vi "TMflexLinkInformation.vi"() -> ()   [LabVIEW 2015]
uses:
  TMflexDatabase.lvclass
  <vilib>/Utility/config.llb/Read Key (String).vi
  <vilib>/addons/database/_DB Variant To Data/Database Variant To Data.xnode
  <vilib>/Utility/config.llb/NI_LVConfig.lvlib
panel:
  out "User Name":string
  in  "Unlink Assembly":T1(radio)=enum."FinalAssembly"
  out "Sql Query":string
  in  "Reset":bool
  out "Link Table":string[][](table)
  in  "Get Link Info":bool
  in  "Stop Button":bool
  in  "Update Link Info":bool
  in  "ExtAssembly":string
  in  "PowerSupply":string
  in  "ChemicalTrap":string
  in  "OxygenSensor":string
  in  "HydrogenSensor":string
  in  "GcAssembly":string
  in  "OcAssembly":string
  in  "PasAssembly":string
  in  "QtmsAssembly":string
  in  "FinalAssembly":string
  # "TMflexLinkInfo: Tools for getting link info, linking and de-linking TMxflex assemblies\nGet Link Info: Scan in the serial number of the desired assembly and click Get Link button\nLink Assembly: Scan in serial numbers of assemblies and click Update Link button\nDe-Link Assembly: Select the unlink radio button and then click Update Link button\nQuit: Hit Stop button"
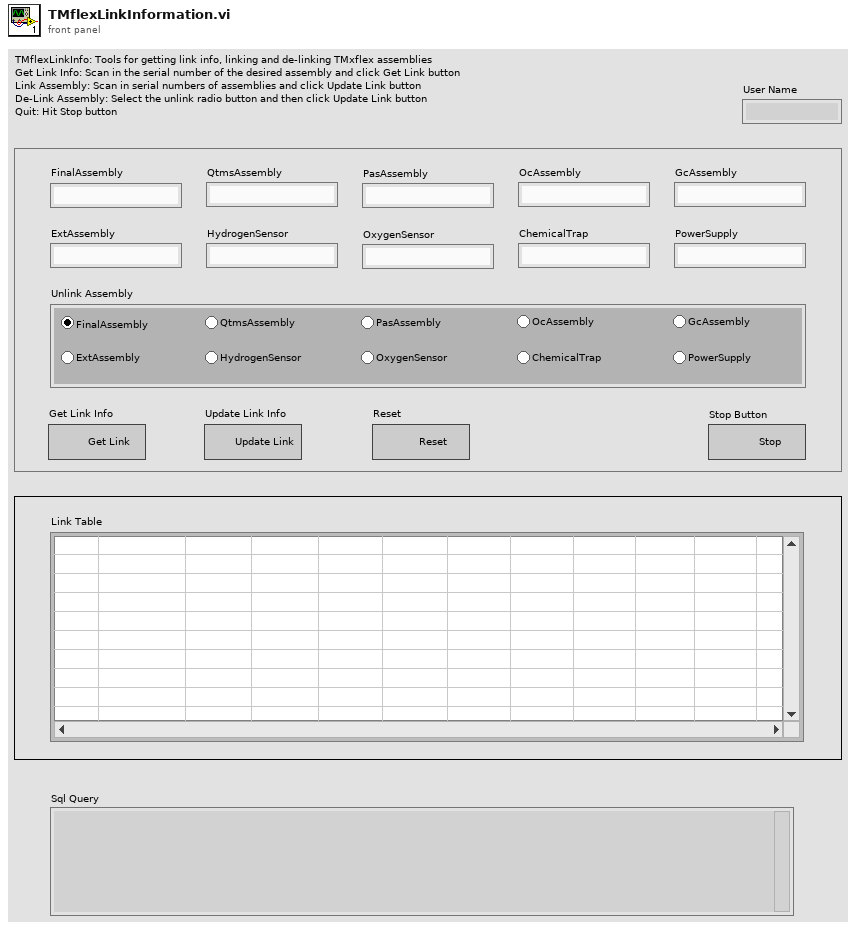
[diagram p1: front panel]
types:
  T1 = enum32{"No Selection", "FinalAssembly", "QtmsAssembly", "PasAssembly", "OcAssembly", "GcAssembly", "ExtAssembly", "HydrogenSensor", "OxygenSensor", "ChemicalTrap", "PowerSupply"}
  T2 = typedef "NI_LVConfig.lvlib/Config Data RefNum.ctl" = refnum<k1>
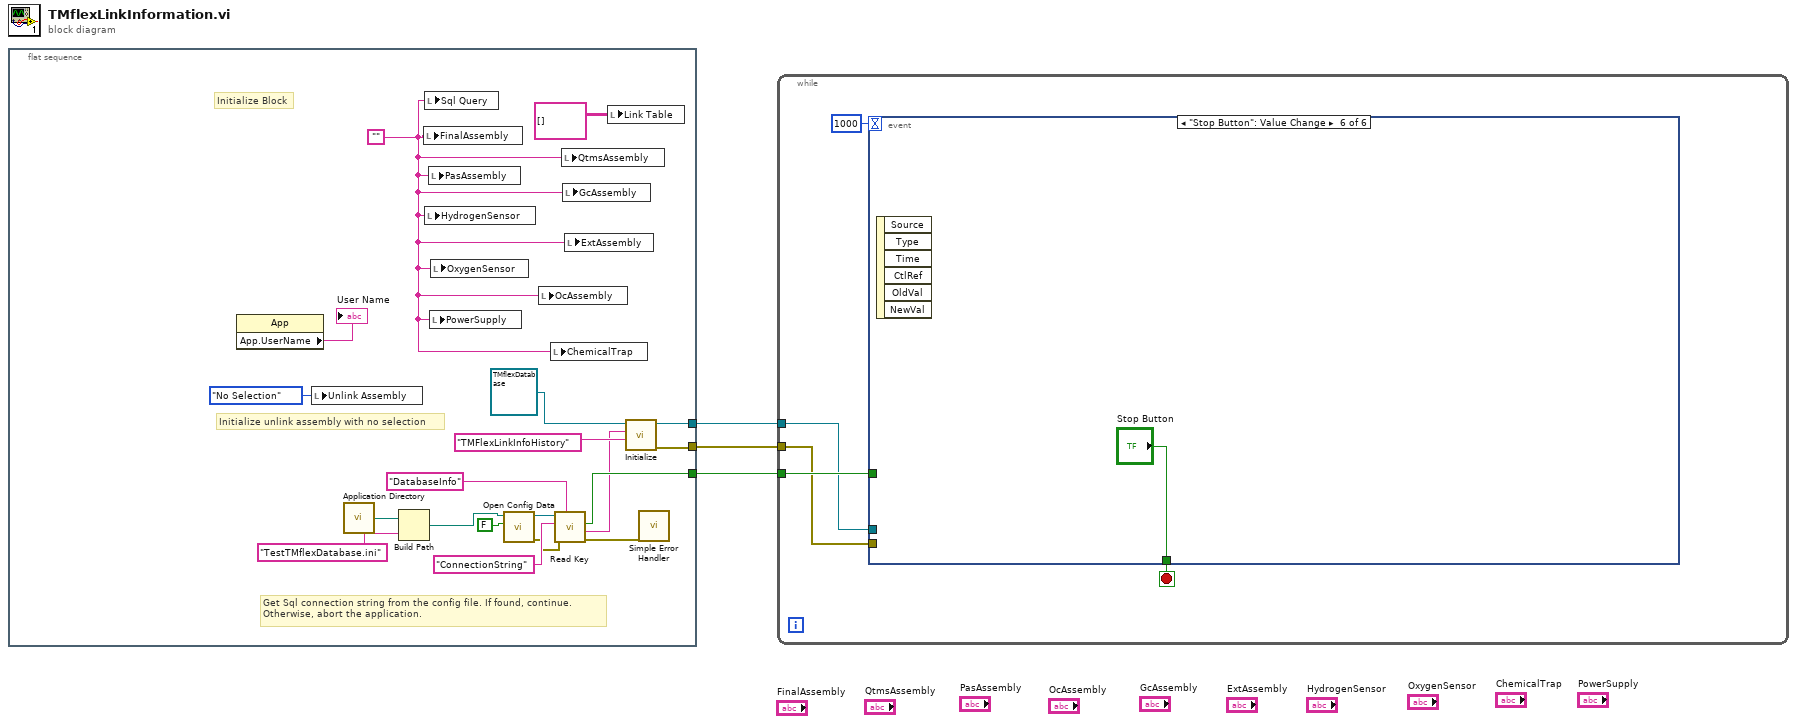
[diagram p0: block diagram]
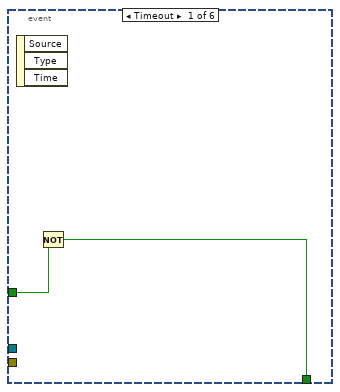
[diagram p2: hidden frame]
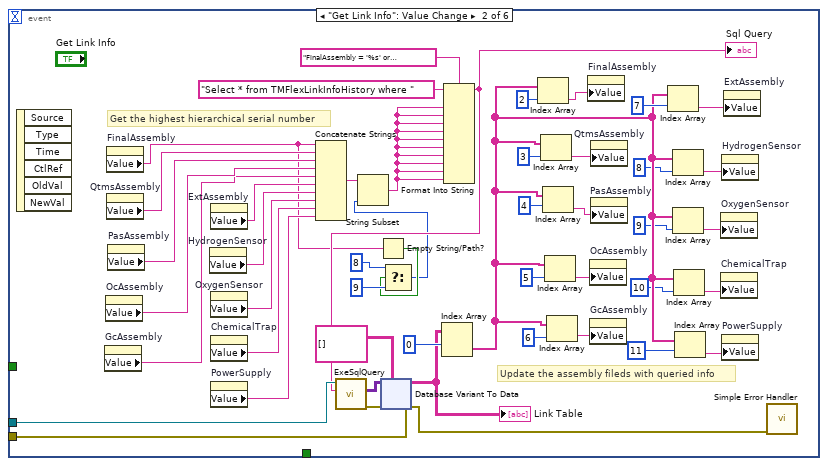
[diagram p3: hidden frame]
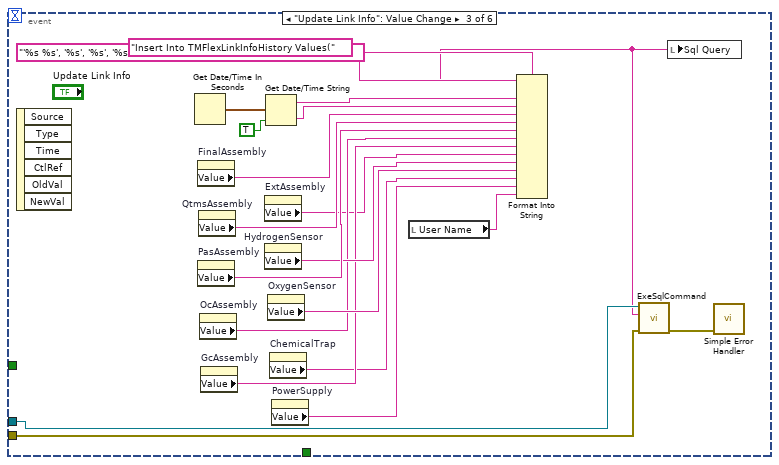
[diagram p4: hidden frame]
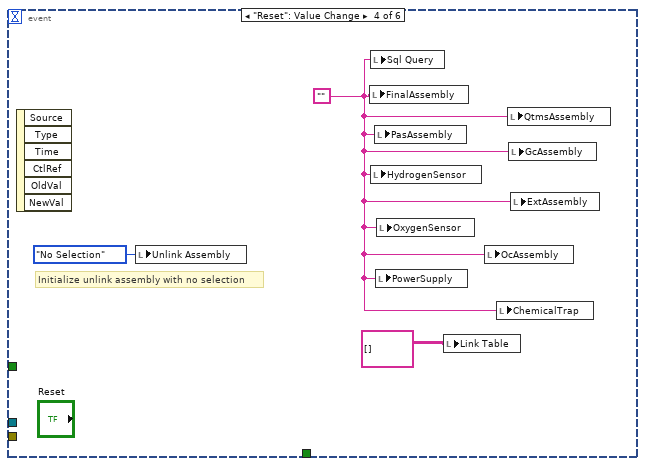
[diagram p5: hidden frame]
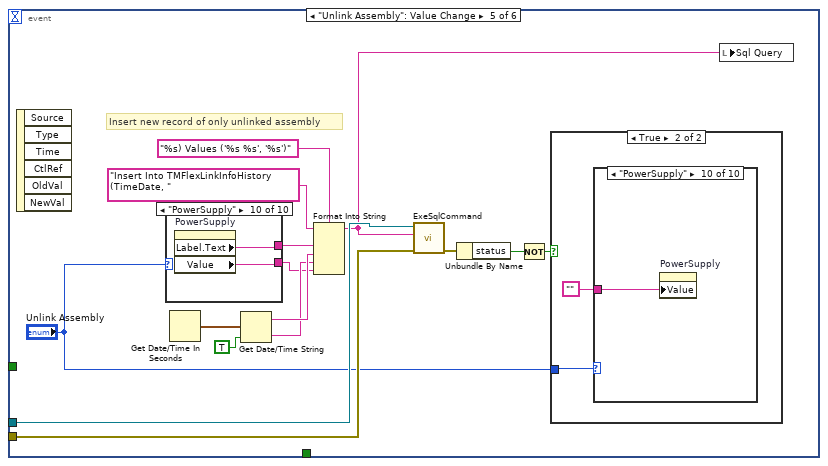
[diagram p6: hidden frame]
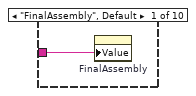
[diagram p8: hidden frame]
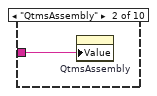
[diagram p9: hidden frame]
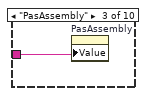
[diagram p10: hidden frame]
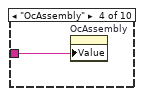
[diagram p11: hidden frame]
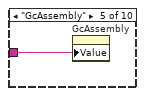
[diagram p12: hidden frame]
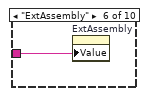
[diagram p13: hidden frame]
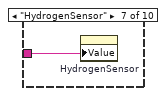
[diagram p14: hidden frame]
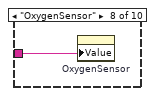
[diagram p15: hidden frame]
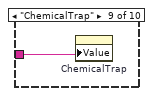
[diagram p16: hidden frame]
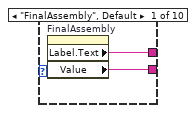
[diagram p17: hidden frame]
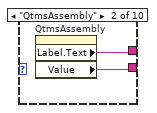
[diagram p18: hidden frame]
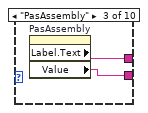
[diagram p19: hidden frame]
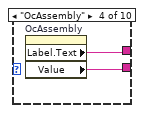
[diagram p20: hidden frame]
diagram:
  n1 = flat-sequence {
    tunnel: [w17] -> w3
    tunnel: [w12] -> w2
    tunnel: [w11] -> w1
    frame #0 {
      w9 = ""
      # "Initialize unlink assembly with no selection"
      # "Initialize Block"
      # "Get Sql connection string from the config file. If found, continue.\nOtherwise, abort the application."
      n2 = property class="App"() -> ("App.UserName"=→"User Name":string)  [unwired: 2 in, 2 out]
      n3 = local write "Unlink Assembly"(T1."No Selection" ("Unlink Assembly")) -> ()
      n4 = call <vilib>:"Application Directory.vi"() -> ("Application Directory"=w6:path)
      n5 = Build Path(base path=w6, name or relative path="TestTMflexDatabase.ini") -> (appended path=w4:path)
      n6 = local write "FinalAssembly"(w9) -> ()
      n7 = local write "Sql Query"(w9) -> ()
      n8 = local write "HydrogenSensor"(w9) -> ()
      n9 = local write "PasAssembly"(w9) -> ()
      n10 = local write "PowerSupply"(w9) -> ()
      n11 = local write "OxygenSensor"(w9) -> ()
      n12 = call <vilib>:"Open Config Data.vi"("create file if necessary (T)"=FALSE, "configuration file path"=w4) -> ("error out"=w16:errorcluster, "refnum"=w21:T2)  [unwired: 7 in, 1 out]
      n13 = local write "OcAssembly"(w9) -> ()
      n14 = local write "ChemicalTrap"(w9) -> ()
      n15 = call-poly <vilib>:"Read Key.vi"("section"="DatabaseInfo", "error in (no error)"=w16, "key"="ConnectionString", "refnum"=w21) -> ("error out"=w18:errorcluster, "value"=w13:string, "found?"=w17:bool)  [unwired: 4 in, 1 out]
      n16 = local write "QtmsAssembly"(w9) -> ()
      n17 = local write "GcAssembly"(w9) -> ()
      n18 = local write "ExtAssembly"(w9) -> ()
      n19 = local write "Link Table"(string[][] []) -> ()
      n20 = call-dynamic "Initialize.vi"("TableName"="TMFlexLinkInfoHistory", "ConnectionString"=w13, "TMflexDatabase in"=refnum<class "TMflexDatabase.lvclass"> refnum ("TMflexDatabase.lvclass")) -> ("error out"=w11:errorcluster, "TMflexDatabase out"=w12:refnum<class "TMflexDatabase.lvclass">)  [unwired: 7 in]
      n21 = call <vilib>:"Simple Error Handler.vi"("error in (no error)"=w18) -> ()  [unwired: 4 in, 5 out]
    }
  }
  n22 = while {
    tunnel: w3 -> [w26]
    tunnel: w2 -> [w23]
    tunnel: w1 -> [w24]
    stop <- w27 stop-if-true
    n23 = event shown="[5] \"Stop Button\": Value Change" {
      selector: _ -> [_ _ _ _ _ _]
      dyn-events: _ -> [_ _ _ _ _ _]
      timeout: 1000 -> [_ _ _ _ _ _]
      tunnel: [w28 _ _ _ _ "Stop Button"] -> w27
      tunnel: w26 -> [w29 _ _ _ _ _]
      tunnel: w24 -> [_ w60 w129 _ w155 _]
      tunnel: w23 -> [_ w59 w130 _ w156 _]
      event Timeout {
        n24 = event-data() -> ()  [unwired: 1 in, 3 out]
        n25 = Not(x=w29) -> (.not. x?=w28:bool)
      }
      event "Get Link Info": Value Change {
        # "Update the assembly fileds with queried info"
        # "Get the highest hierarchical serial number"
        n26 = event-data() -> ()  [unwired: 1 in, 6 out]
        n27 = property on="GcAssembly" class="Str"() -> ("Value"=w73:string)  [unwired: 2 in, 2 out]
        n28 = property on="OcAssembly" class="Str"() -> ("Value"=w74:string)  [unwired: 2 in, 2 out]
        n29 = property on="FinalAssembly" class="Str"() -> ("Value"=w30:string)  [unwired: 2 in, 2 out]
        n30 = property on="QtmsAssembly" class="Str"() -> ("Value"=w76:string)  [unwired: 2 in, 2 out]
        n31 = property on="PasAssembly" class="Str"() -> ("Value"=w75:string)  [unwired: 2 in, 2 out]
        n32 = property on="HydrogenSensor" class="Str"() -> ("Value"=w71:string)  [unwired: 2 in, 2 out]
        n33 = property on="ExtAssembly" class="Str"() -> ("Value"=w72:string)  [unwired: 2 in, 2 out]
        n34 = property on="OxygenSensor" class="Str"() -> ("Value"=w70:string)  [unwired: 2 in, 2 out]
        n35 = property on="ChemicalTrap" class="Str"() -> ("Value"=w69:string)  [unwired: 2 in, 2 out]
        n36 = property on="PowerSupply" class="Str"() -> ("Value"=w68:string)  [unwired: 2 in, 2 out]
        n37 = Concatenate Strings(w30, w76, w75, w74, w73, w72, w71, w70, w69, w68) -> (w67:string)
        n38 = Empty String/Path?(string/path=w30) -> (empty?=w32:bool)
        n39 = Select(t=8, s=w32, f=9) -> (s? t:f=w31:i32)
        n40 = String Subset(string=w67, length (rest)=w31) -> (substring=w65:string)  [unwired: 1 in]
        n41 = Format Into String(format string="FinalAssembly = '%s' or  QtmsAssembly = '%s' or PasAssembly = '%s' or OcAssembly = '%s' or GcAssembly = '%s' or ExtAssembly = '%s' or HydrogenSensor = '%s' or OxygenSensor = '%s' or ChemicalTrap = '%s' or PowerSupply = '%s' Order by TimeDate Desc ", initial string="Select * from TMFlexLinkInfoHistory where ", w65, w65, w65, w65, w65, w65, w65, w65, w65, w65) -> (resulting string=w35:string)  [unwired: 1 in, 1 out]
        "Sql Query" <- w35
        n42 = call-dynamic "ExeSqlQuery.vi"("error in (no error)"=w60, "SqlQuery"=w35, "TMflexDatabase in"=w59) -> ("error out"=w62:errorcluster, "data"=w64:variant[][])  [unwired: 6 in, 1 out]
        n43 = xnode "Database Variant To Data"("database variant"=w64, "error in (no error)"=w62, "type"=string[][] []) -> ("data"=w36:string[][], "error out"=w61:errorcluster)
        "Link Table" <- w36
        n44 = Index Array(array=w36, index (row)=0 ("index")) -> (element=w44:string[])  [unwired: 1 in]
        n45 = Index Array(array=w44, index=2) -> (element=w56:string)
        n46 = Index Array(array=w44, index=3) -> (element=w51:string)
        n47 = Index Array(array=w44, index=4) -> (element=w50:string)
        n48 = Index Array(array=w44, index=5) -> (element=w49:string)
        n49 = Index Array(array=w44, index=6) -> (element=w48:string)
        n50 = property on="FinalAssembly" class="Str"("Value"=w56) -> ()  [unwired: 2 in, 2 out]
        n51 = property on="OcAssembly" class="Str"("Value"=w49) -> ()  [unwired: 2 in, 2 out]
        n52 = property on="GcAssembly" class="Str"("Value"=w48) -> ()  [unwired: 2 in, 2 out]
        n53 = property on="QtmsAssembly" class="Str"("Value"=w51) -> ()  [unwired: 2 in, 2 out]
        n54 = property on="PasAssembly" class="Str"("Value"=w50) -> ()  [unwired: 2 in, 2 out]
        n55 = Index Array(array=w44, index=7) -> (element=w47:string)
        n56 = Index Array(array=w44, index=8) -> (element=w45:string)
        n57 = Index Array(array=w44, index=9) -> (element=w39:string)
        n58 = Index Array(array=w44, index=10) -> (element=w38:string)
        n59 = Index Array(array=w44, index=11) -> (element=w37:string)
        n60 = property on="OxygenSensor" class="Str"("Value"=w39) -> ()  [unwired: 2 in, 2 out]
        n61 = property on="ChemicalTrap" class="Str"("Value"=w38) -> ()  [unwired: 2 in, 2 out]
        n62 = property on="HydrogenSensor" class="Str"("Value"=w45) -> ()  [unwired: 2 in, 2 out]
        n63 = property on="PowerSupply" class="Str"("Value"=w37) -> ()  [unwired: 2 in, 2 out]
        n64 = property on="ExtAssembly" class="Str"("Value"=w47) -> ()  [unwired: 2 in, 2 out]
        n65 = call <vilib>:"Simple Error Handler.vi"("error in (no error)"=w61) -> ()  [unwired: 4 in, 5 out]
      }
      event "Update Link Info": Value Change {
        n66 = event-data() -> ()  [unwired: 1 in, 6 out]
        n67 = Get Date/Time In Seconds() -> (seconds since 1Jan1904=w141:timestamp)
        n68 = property on="FinalAssembly" class="Str"() -> ("Value"=w136:string)  [unwired: 2 in, 2 out]
        n69 = property on="PasAssembly" class="Str"() -> ("Value"=w134:string)  [unwired: 2 in, 2 out]
        n70 = property on="QtmsAssembly" class="Str"() -> ("Value"=w135:string)  [unwired: 2 in, 2 out]
        n71 = property on="OcAssembly" class="Str"() -> ("Value"=w128:string)  [unwired: 2 in, 2 out]
        n72 = property on="GcAssembly" class="Str"() -> ("Value"=w127:string)  [unwired: 2 in, 2 out]
        n73 = property on="ExtAssembly" class="Str"() -> ("Value"=w126:string)  [unwired: 2 in, 2 out]
        n74 = property on="HydrogenSensor" class="Str"() -> ("Value"=w133:string)  [unwired: 2 in, 2 out]
        n75 = Get Date/Time String(seconds (now)=w141, want seconds? (F)=TRUE) -> (date string=w138:string, time string=w137:string)  [unwired: 1 in]
        n76 = property on="OxygenSensor" class="Str"() -> ("Value"=w132:string)  [unwired: 2 in, 2 out]
        n77 = property on="ChemicalTrap" class="Str"() -> ("Value"=w125:string)  [unwired: 2 in, 2 out]
        n78 = property on="PowerSupply" class="Str"() -> ("Value"=w124:string)  [unwired: 2 in, 2 out]
        n79 = local read "User Name"() -> (w122:string)
        n80 = Format Into String(format string="'%s %s', '%s', '%s', '%s', '%s', '%s', '%s', '%s', '%s', '%s', '%s', '%s')", initial string="Insert Into TMFlexLinkInfoHistory Values(", w138, w137, w136, w135, w134, w128, w127, w126, w133, w132, w125, w124, w122) -> (resulting string=w123:string)  [unwired: 1 in, 1 out]
        n81 = call-dynamic "ExeSqlCommand.vi"("error in (no error)"=w129, "SqlCommand"=w123, "TMflexDatabase in"=w130) -> ("error out"=w131:errorcluster)  [unwired: 7 in, 1 out]
        n82 = local write "Sql Query"(w123) -> ()
        n83 = call <vilib>:"Simple Error Handler.vi"("error in (no error)"=w131) -> ()  [unwired: 4 in, 5 out]
      }
      event "Reset": Value Change {
        w143 = ""
        # "Initialize unlink assembly with no selection"
        n84 = event-data() -> ()  [unwired: 1 in, 6 out]
        n85 = local write "Unlink Assembly"(T1."No Selection" ("Unlink Assembly")) -> ()
        n86 = local write "FinalAssembly"(w143) -> ()
        n87 = local write "Sql Query"(w143) -> ()
        n88 = local write "HydrogenSensor"(w143) -> ()
        n89 = local write "PasAssembly"(w143) -> ()
        n90 = local write "PowerSupply"(w143) -> ()
        n91 = local write "OxygenSensor"(w143) -> ()
        n92 = local write "Link Table"(string[][] []) -> ()
        n93 = local write "OcAssembly"(w143) -> ()
        n94 = local write "ChemicalTrap"(w143) -> ()
        n95 = local write "QtmsAssembly"(w143) -> ()
        n96 = local write "GcAssembly"(w143) -> ()
        n97 = local write "ExtAssembly"(w143) -> ()
      }
      event "Unlink Assembly": Value Change {
        # "Insert new record of only unlinked assembly"
        n98 = event-data() -> ()  [unwired: 1 in, 6 out]
        n99 = case shown="\"PowerSupply\"" "Unlink Assembly" {
          tunnel: [w174 w176 w178 w180 w182 w184 w186 w188 w190 w192] -> w152
          tunnel: [w173 w175 w177 w179 w181 w183 w185 w187 w189 w191] -> w149
          frame "FinalAssembly", Default {
            n100 = property on="FinalAssembly" class="Str"() -> ("Label.Text"=w174:string, "Value"=w173:string)  [unwired: 2 in, 2 out]
          }
          frame "QtmsAssembly" {
            n101 = property on="QtmsAssembly" class="Str"() -> ("Label.Text"=w176:string, "Value"=w175:string)  [unwired: 2 in, 2 out]
          }
          frame "PasAssembly" {
            n102 = property on="PasAssembly" class="Str"() -> ("Label.Text"=w178:string, "Value"=w177:string)  [unwired: 2 in, 2 out]
          }
          frame "OcAssembly" {
            n103 = property on="OcAssembly" class="Str"() -> ("Label.Text"=w180:string, "Value"=w179:string)  [unwired: 2 in, 2 out]
          }
          frame "GcAssembly" {
            n104 = property on="GcAssembly" class="Str"() -> ("Label.Text"=w182:string, "Value"=w181:string)  [unwired: 2 in, 2 out]
          }
          frame "ExtAssembly" {
            n105 = property on="ExtAssembly" class="Str"() -> ("Label.Text"=w184:string, "Value"=w183:string)  [unwired: 2 in, 2 out]
          }
          frame "HydrogenSensor" {
            n106 = property on="HydrogenSensor" class="Str"() -> ("Label.Text"=w186:string, "Value"=w185:string)  [unwired: 2 in, 2 out]
          }
          frame "OxygenSensor" {
            n107 = property on="OxygenSensor" class="Str"() -> ("Label.Text"=w188:string, "Value"=w187:string)  [unwired: 2 in, 2 out]
          }
          frame "ChemicalTrap" {
            n108 = property on="ChemicalTrap" class="Str"() -> ("Label.Text"=w190:string, "Value"=w189:string)  [unwired: 2 in, 2 out]
          }
          frame "PowerSupply" {
            n109 = property on="PowerSupply" class="Str"() -> ("Label.Text"=w192:string, "Value"=w191:string)  [unwired: 2 in, 2 out]
          }
        }
        n110 = Get Date/Time In Seconds() -> (seconds since 1Jan1904=w158:timestamp)
        n111 = Get Date/Time String(seconds (now)=w158, want seconds? (F)=TRUE) -> (date string=w151:string, time string=w150:string)  [unwired: 1 in]
        n112 = Format Into String(format string="%s) Values ('%s %s', '%s')", initial string="Insert Into TMFlexLinkInfoHistory (TimeDate, ", w152, w151, w150, w149) -> (resulting string=w146:string)  [unwired: 1 in, 1 out]
        n113 = call-dynamic "ExeSqlCommand.vi"("error in (no error)"=w155, "SqlCommand"=w146, "TMflexDatabase in"=w156) -> ("error out"=w154:errorcluster)  [unwired: 7 in, 1 out]
        n114 = Unbundle By Name(w154) -> ("status"=w147:bool)
        n115 = Not(x=w147) -> (.not. x?=w148:bool)
        n116 = case shown="True" w148 {
          tunnel: "Unlink Assembly" -> [_ w162]
          frame False {
          }
          frame True {
            n117 = case shown="\"PowerSupply\"" w162 {
              tunnel: "" -> [w163 w164 w165 w166 w167 w168 w169 w170 w171 w172]
              frame "FinalAssembly", Default {
                n118 = property on="FinalAssembly" class="Str"("Value"=w163) -> ()  [unwired: 2 in, 2 out]
              }
              frame "QtmsAssembly" {
                n119 = property on="QtmsAssembly" class="Str"("Value"=w164) -> ()  [unwired: 2 in, 2 out]
              }
              frame "PasAssembly" {
                n120 = property on="PasAssembly" class="Str"("Value"=w165) -> ()  [unwired: 2 in, 2 out]
              }
              frame "OcAssembly" {
                n121 = property on="OcAssembly" class="Str"("Value"=w166) -> ()  [unwired: 2 in, 2 out]
              }
              frame "GcAssembly" {
                n122 = property on="GcAssembly" class="Str"("Value"=w167) -> ()  [unwired: 2 in, 2 out]
              }
              frame "ExtAssembly" {
                n123 = property on="ExtAssembly" class="Str"("Value"=w168) -> ()  [unwired: 2 in, 2 out]
              }
              frame "HydrogenSensor" {
                n124 = property on="HydrogenSensor" class="Str"("Value"=w169) -> ()  [unwired: 2 in, 2 out]
              }
              frame "OxygenSensor" {
                n125 = property on="OxygenSensor" class="Str"("Value"=w170) -> ()  [unwired: 2 in, 2 out]
              }
              frame "ChemicalTrap" {
                n126 = property on="ChemicalTrap" class="Str"("Value"=w171) -> ()  [unwired: 2 in, 2 out]
              }
              frame "PowerSupply" {
                n127 = property on="PowerSupply" class="Str"("Value"=w172) -> ()  [unwired: 2 in, 2 out]
              }
            }
          }
        }
        n128 = local write "Sql Query"(w146) -> ()
      }
      event "Stop Button": Value Change {
        n129 = event-data() -> ()  [unwired: 1 in, 6 out]
      }
    }
  }
